vi "Stop.vi"(8 "error in (no error)":errorcluster, 11 "Panel State Data In":T1) -> (0 "error out":errorcluster, 3 "Panel State Data Out":T1)   [LabVIEW 2025]
uses:
  Typedef/Test Panel State Data.ctl
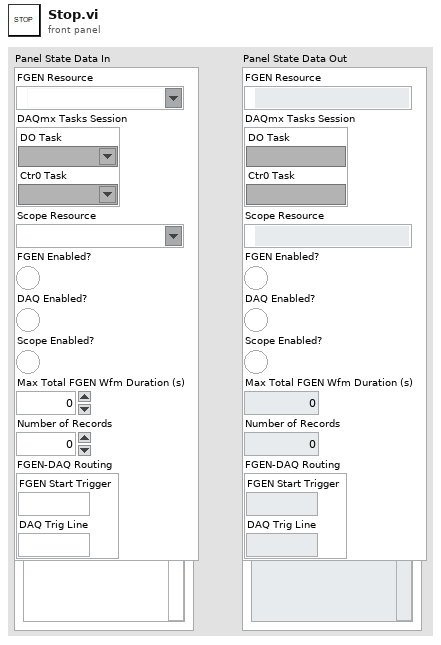
[diagram p1: front panel]
types:
  T1 = typedef "Test Panel State Data.ctl" = cluster{"FGEN Resource":refnum<k15>, "DAQmx Tasks Session":cluster{"DO Task":refnum<k21>, "Ctr0 Task":refnum<k21>}, "Scope Resource":refnum<k15>, "FGEN Enabled?":bool, "DAQ Enabled?":bool, "Scope Enabled?":bool, "Max Total FGEN Wfm Duration (s)":dbl, "Number of Records":i32, "FGEN-DAQ Routing":cluster{"FGEN Start Trigger":string, "DAQ Trig Line":string}}
  T2 = cluster{"DO Task":refnum<k21>, "Ctr0 Task":refnum<k21>}
  T3 = cluster{"FGEN Start Trigger":string, "DAQ Trig Line":string}
  T4 = enum16{"Reset", "Start", "Read", "Pause", "Resume"}
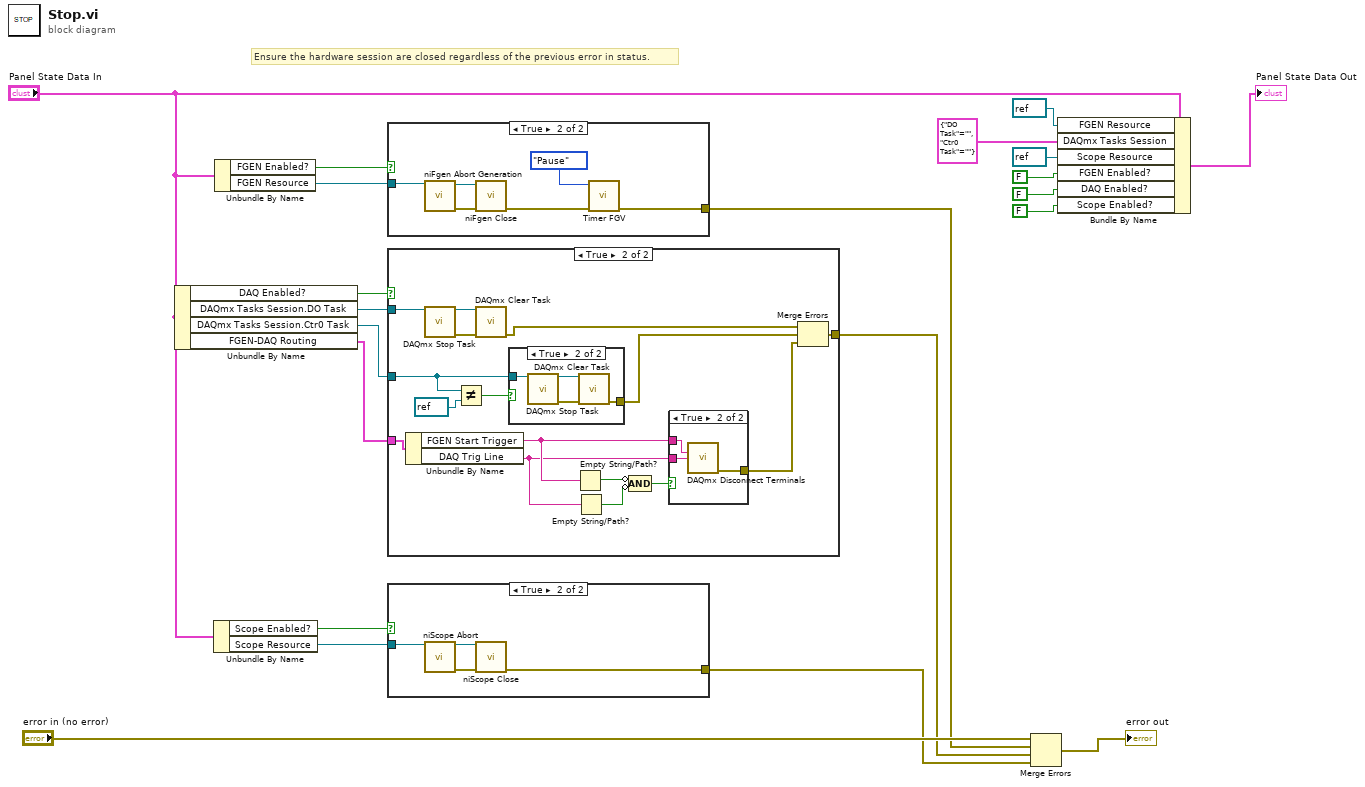
[diagram p0: block diagram]
diagram:
  # "Ensure the hardware session are closed regardless of the previous error in status."
  n1 = Unbundle By Name("Panel State Data In") -> ("DAQ Enabled?"=w17:bool, "DAQmx Tasks Session.DO Task"=w18:refnum<k21>, "DAQmx Tasks Session.Ctr0 Task"=w3:refnum<k21>, "FGEN-DAQ Routing"=w1:T3)
  n2 = Unbundle By Name("Panel State Data In") -> ("Scope Enabled?"=w16:bool, "Scope Resource"=w15:refnum<k15>)
  n3 = Unbundle By Name("Panel State Data In") -> ("FGEN Enabled?"=w20:bool, "FGEN Resource"=w19:refnum<k15>)
  n4 = case shown="True" w20 {
    tunnel: w19 -> [_ w27]
    tunnel: [_ w23] -> w12
    frame False {
    }
    frame True {
      n5 = call <instrlib>:"niFgen Abort Generation.vi"("Instrument Handle"=w27) -> ("error out"=w25:errorcluster, "Instrument Handle Out"=w26:refnum<k15>)  [unwired: 9 in]
      n6 = call <instrlib>:"niFgen Close.vi"("error in (no error)"=w25, "Instrument Handle"=w26) -> ("error out"=w24:errorcluster)  [unwired: 9 in]
      n7 = call "Timer FGV.vi"("error in (no error)"=w24, "Timer mode"=T4."Pause") -> ("error out"=w23:errorcluster)  [unwired: 6 in, 3 out]
    }
  }
  n8 = case shown="True" w17 {
    tunnel: w18 -> [_ w43]
    tunnel: [_ w34] -> w11
    tunnel: w3 -> [_ w30]
    tunnel: w1 -> [_ w39]
    frame False {
    }
    frame True {
      n9 = Unbundle By Name(w39) -> ("FGEN Start Trigger"=w36:string, "DAQ Trig Line"=w35:string)
      n10 = call <vilib>:"DAQmx Stop Task.vi"("task/channels in"=w43) -> ("task out"=w42:refnum<k21>, "error out"=w41:errorcluster)  [unwired: 13 in]
      n11 = Not Equal?(x=w30, y=refnum<k21> refnum) -> (x != y?=w28:bool)
      n12 = call <vilib>:"DAQmx Clear Task.vi"("task in"=w42, "error in"=w41) -> ("error out"=w33:errorcluster)  [unwired: 13 in]
      n13 = case shown="True" w28 {
        tunnel: [_ w45] -> w40
        tunnel: w30 -> [_ w44]
        frame False {
        }
        frame True {
          n14 = call <vilib>:"DAQmx Stop Task.vi"("task/channels in"=w44) -> ("task out"=w46:refnum<k21>, "error out"=w47:errorcluster)  [unwired: 13 in]
          n15 = call <vilib>:"DAQmx Clear Task.vi"("task in"=w46, "error in"=w47) -> ("error out"=w45:errorcluster)  [unwired: 13 in]
        }
      }
      n16 = Empty String/Path?(string/path=w36) -> (empty?=w38:bool)
      n17 = Empty String/Path?(string/path=w35) -> (empty?=w37:bool)
      n18 = Compound Arithmetic op=AND(invert w38, invert w37) -> (w31:bool)
      n19 = case shown="True" w31 {
        tunnel: w36 -> [_ w50]
        tunnel: w35 -> [_ w49]
        tunnel: [_ w48] -> w32
        frame False {
        }
        frame True {
          n20 = call <vilib>:"DAQmx Disconnect Terminals.vi"("source terminal"=w50, "destination terminal"=w49) -> ("error out"=w48:errorcluster)  [unwired: 13 in]
        }
      }
      n21 = Merge Errors(w33, w40, w32) -> (w34:errorcluster)
    }
  }
  n22 = case shown="True" w16 {
    tunnel: w15 -> [_ w51]
    tunnel: [_ w52] -> w10
    frame False {
    }
    frame True {
      n23 = call <instrlib>:"niScope Abort.vi"("instrument handle"=w51) -> ("instrument handle out"=w54:refnum<k15>, "error out"=w53:errorcluster)  [unwired: 13 in]
      n24 = call <instrlib>:"niScope Close.vi"("instrument handle"=w54, "error in"=w53) -> ("error out"=w52:errorcluster)  [unwired: 13 in]
    }
  }
  n25 = Merge Errors("error in (no error)", w12, w11, w10) -> (→"error out":errorcluster)
  n26 = Bundle By Name(cluster="Panel State Data In", "FGEN Resource"=refnum<k15> refnum, "DAQmx Tasks Session"=T2 {"DO Task"="", "Ctr0 Task"=""}, "Scope Resource"=refnum<k15> refnum, "FGEN Enabled?"=FALSE, "DAQ Enabled?"=FALSE, "Scope Enabled?"=FALSE) -> (→"Panel State Data Out":T1)
